vi "APU 1.0 In Place Input Write Structure.vi"(5 "Device Inputs":dbl[](array[numeric]), 7 "Last Device Inputs":dbl[](array[numeric]), 8 "error in (no error)":errorcluster, 9 "FPGA ref in":T1, 11 "1.0 APU in":T4={"register names"={"shared settings"="", "input"="", "settings"="", "output"=""}, "shared settings"={"cycle start"=0.0, "crank start"=0, "stuck limit"=0.0}, "settings"={"acceleration"=0.0, "max cycle"=0.0, "enable accel"=FALSE}, "FIFO indexes"={"inputs"={"desired speed"=0, "reset"=0}, "outputs"={"crank angle"=0, "cycle angle"=0, "actual speed"=0}}, "input"={"desired speed"=0.0, "reset"=TRUE}, "degrees of 1 cycle u16"=0.0, "degrees of 1 crank u16"=0.0} {"shared settings"."cycle start" format="%#.15g"}) -> (0 "error out":errorcluster, 1 "FPGA ref out":T1, 3 "1.0 APU out":T4={"register names"={"shared settings"="", "input"="", "settings"="", "output"=""}, "shared settings"={"cycle start"=0.0, "crank start"=0, "stuck limit"=0.0}, "settings"={"acceleration"=0.0, "max cycle"=0.0, "enable accel"=FALSE}, "FIFO indexes"={"inputs"={"desired speed"=0, "reset"=0}, "outputs"={"crank angle"=0, "cycle angle"=0, "actual speed"=0}}, "input"={"desired speed"=0.0, "reset"=TRUE}, "degrees of 1 cycle u16"=0.0, "degrees of 1 crank u16"=0.0} {"shared settings"."cycle start" format="%#.15g"})   [LabVIEW 2020, in "Engine Simulation Toolkit Engine.lvlib"]
uses:
  Engine Simulation Toolkit Engine.lvlib
  Shared/1.0 APU Engine Data.ctl
  Shared/1.0 APU Engine FIFO Idxs.ctl
  APU 1.0 Run Refs.ctl
  APU 1.0 Output Ref.ctl
  APU 1.0 Input Ref.ctl
  Shared/DBL Speed to FXP.vi
  APU 1.0 FPGA Inputs Write Node.vi
  Shared/Engine Simulation Toolkit Shared.lvlib
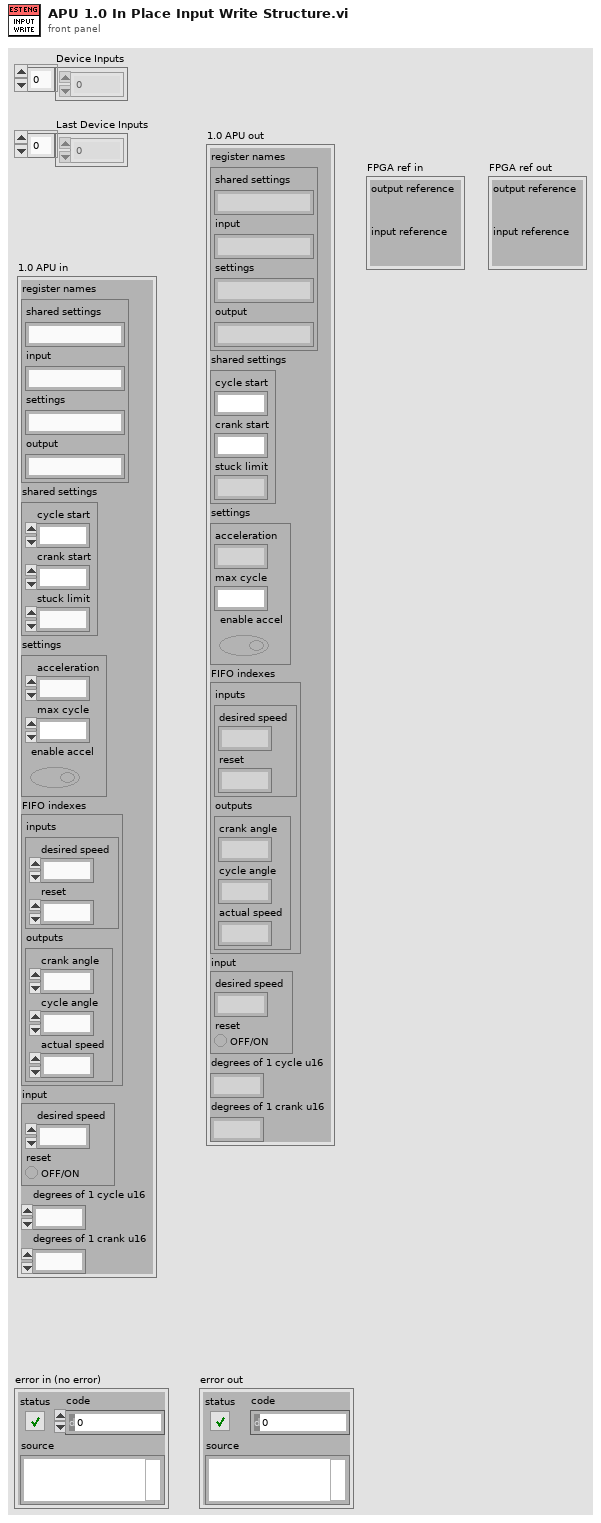
[diagram p1: front panel]
types:
  T1 = typedef "Engine Simulation Toolkit Engine.lvlib/APU 1.0 Run Refs.ctl" = cluster{"output reference":T2, "input reference":T3}
  T2 = typedef "Engine Simulation Toolkit Engine.lvlib/APU 1.0 Output Ref.ctl" = refnum<k20>
  T3 = typedef "Engine Simulation Toolkit Engine.lvlib/APU 1.0 Input Ref.ctl" = refnum<k20>
  T4 = typedef "Engine Simulation Toolkit Shared.lvlib/1.0 APU Engine Data.ctl" = cluster{"register names":cluster{"shared settings":string, "input":string, "settings":string, "output":string}, "shared settings":cluster{"cycle start":fxp<+,2,2>, "crank start":u16, "stuck limit":fxp<+,18,18>}, "settings":cluster{"acceleration":fxp<+,18,-20>, "max cycle":fxp<+,2,2>, "enable accel":bool}, "FIFO indexes":T5, "input":cluster{"desired speed":fxp<+/-,23,2>, "reset":bool}, "degrees of 1 cycle u16":dbl, "degrees of 1 crank u16":dbl}
  T5 = typedef "Engine Simulation Toolkit Shared.lvlib/1.0 APU Engine FIFO Idxs.ctl" = cluster{"inputs":cluster{"desired speed":i32, "reset":i32}, "outputs":cluster{"crank angle":i32, "cycle angle":i32, "actual speed":i32}}
  T6 = cluster{"desired speed":fxp<+/-,23,2>, "reset":bool}
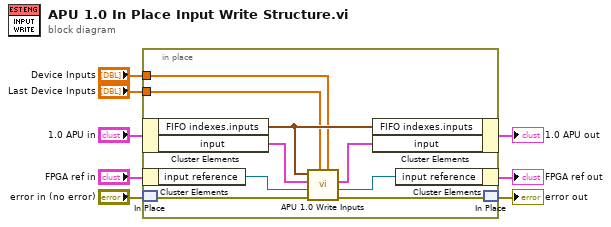
[diagram p0: block diagram]
diagram:
  n1 = in-place {
    in-place-border: "Last Device Inputs" -> [w12]
    in-place-border: "Device Inputs" -> [w11]
    n2 = in-place-cluster #1("1.0 APU in") -> ("FIFO indexes.inputs"=w14:cluster{"desired speed":i32, "reset":i32}, "input"=w15:T6)
    n3 = in-place-cluster #2("FPGA ref in") -> ("input reference"=w10:T3)
    n4 = in-place-match #3("error in (no error)") -> (w17:errorcluster)
    n5 = call "APU 1.0 Write Inputs.vi"("Device inputs"=w11, "Last Device inputs"=w12, "error in (no error)"=w17, "input reference in"=w10, "input in"=w15, "FIFO indexes.inputs"=w14) -> ("error out"=w16:errorcluster, "input reference out"=w9:T3, "input out"=w13:T6)  [unwired: 3 in]
    n6 = in-place-cluster #1("FIFO indexes.inputs"=w14, "input"=w13) -> (→"1.0 APU out":T4)
    n7 = in-place-cluster #2("input reference"=w9) -> (→"FPGA ref out":T1)
    n8 = in-place-match #3(w16) -> (→"error out":errorcluster)
  }
